vi "getLow2bitNumber.vi"(11 "number":u16) -> (2 "outputNum":u8)   [LabVIEW 2016]
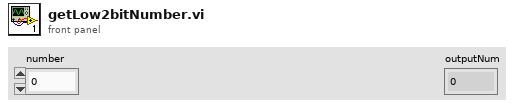
[diagram p1: front panel]
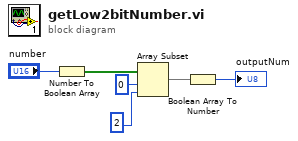
[diagram p0: block diagram]
diagram:
  n1 = Number To Boolean Array(number="number") -> (Boolean array=w6:bool[])
  n2 = Array Subset(array=w6, index=0, length=2) -> (w3:bool[])
  n3 = Boolean Array To Number(Boolean array=w3) -> (number=→"outputNum":u32)
